vi "Modbus LDO Boolean Decode.vi"(8 "error in":errorcluster, 11 "PLC Data":T1 {"PLC Data - LDO"."Timing"."Absolute Time" format="%<%H:%M:%S%3u>t"; "PLC Data - LDO"."Timing"."Display Time" format="%#.20f"; "PLC Data - LDO"."Timing"."Test Time Ref" format="%#.20f"; "PLC Data - LDO"."Timing"."Precondition Time Ref" format="%#.20f"; "PLC Data - LDO"."Timing"."First Call Time Ref" format="%#.20f"; "PLC Data - FVIR"."Timing"."Absolute Time" format="%<%H:%M:%S%3u>t"; "PLC Data - FVIR"."Timing"."Display Time" format="%#.20f"; "PLC Data - FVIR"."Timing"."Test Time Ref" format="%#.20f"; "PLC Data - FVIR"."Timing"."Precondition Time Ref" format="%#.20f"; "PLC Data - FVIR"."Timing"."First Call Time Ref" format="%#.20f"}) -> (0 "error out":errorcluster, 3 "PLC Data Out":T1 {"PLC Data - LDO"."Timing"."Absolute Time" format="%<%H:%M:%S%3u>t"; "PLC Data - LDO"."Timing"."Display Time" format="%#.20f"; "PLC Data - LDO"."Timing"."Test Time Ref" format="%#.20f"; "PLC Data - LDO"."Timing"."Precondition Time Ref" format="%#.20f"; "PLC Data - LDO"."Timing"."First Call Time Ref" format="%#.20f"; "PLC Data - FVIR"."Timing"."Absolute Time" format="%<%H:%M:%S%3u>t"; "PLC Data - FVIR"."Timing"."Display Time" format="%#.20f"; "PLC Data - FVIR"."Timing"."Test Time Ref" format="%#.20f"; "PLC Data - FVIR"."Timing"."Precondition Time Ref" format="%#.20f"; "PLC Data - FVIR"."Timing"."First Call Time Ref" format="%#.20f"})   [LabVIEW 2023, in "Modbus.lvlib"]
uses:
  Modbus.lvlib
  Modbus PLC Data All.ctl
  Modbus FVIR Control.ctl
  Modbus Timing.ctl
  <vilib>/Utility/miscctls.llb/LVDateTimeRec.ctl
  Modbus LDO Control.ctl
  WritingDataFile/Data to Save.ctl
  support/Terminate Conditions Cluster.ctl
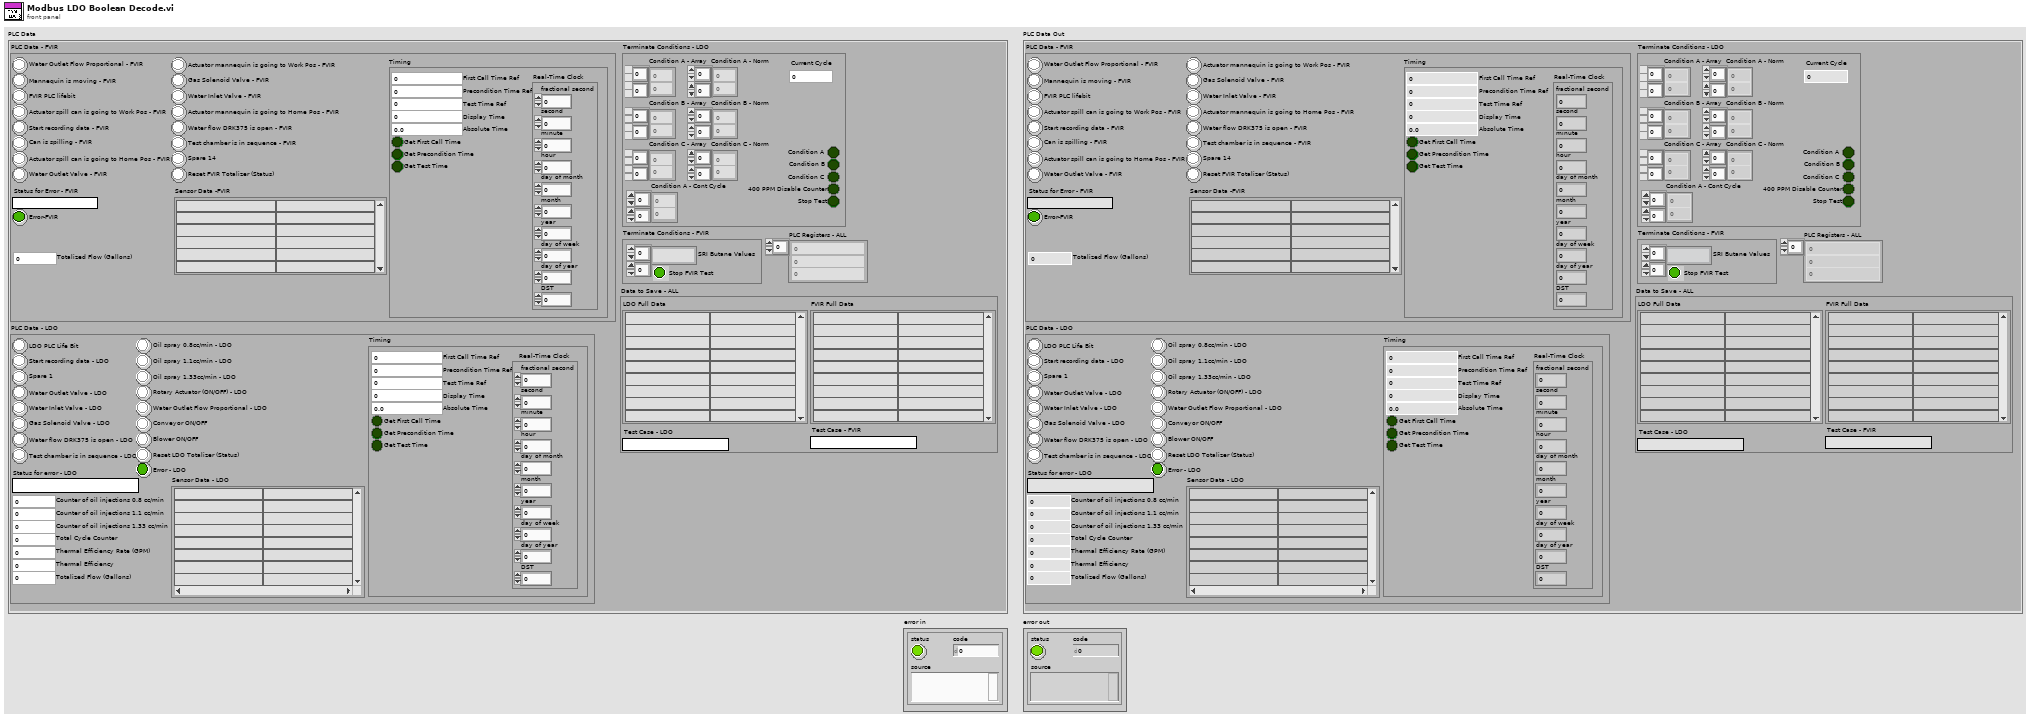
[diagram p1: front panel]
types:
  T1 = typedef "Modbus PLC Data All.ctl" = cluster{"PLC Data - FVIR":T2, "PLC Data - LDO":T5, "PLC Registers - ALL":i16[], "Data to Save - ALL":T6, "Terminate Conditions - LDO":T7, "Terminate Conditions - FVIR":cluster{"SRI Butane Values":string[][], "Stop FVIR Test":bool}}
  T2 = typedef "Modbus FVIR Control.ctl" = cluster{"Reset FVIR Totalizer (Status)":bool, "Spare 14":bool, "Actuator mannequin is going to Work Pos - FVIR":bool, "Actuator mannequin is going to Home Pos - FVIR":bool, "Test chamber is in sequence - FVIR ":bool, "Water flow DRK375 is open - FVIR":bool, "Gas Solenoid Valve - FVIR":bool, "Water Inlet Valve - FVIR":bool, "Water Outlet Flow Proportional - FVIR":bool, "Start recording data - FVIR":bool, "Actuator spill can is going to Work Pos - FVIR":bool, "Actuator spill can is going to Home Pos - FVIR":bool, "Water Outlet Valve - FVIR":bool, "Can is spilling - FVIR":bool, "Mannequin is moving - FVIR":bool, "FVIR PLC lifebit":bool, "Status for Error - FVIR":string, "Error-FVIR":bool, "Sensor Data -FVIR":string[][], "Totalized Flow (Gallons)":dbl, "Timing":T3}
  T3 = typedef "Modbus Timing.ctl" = cluster{"First Call Time Ref":dbl, "Precondition Time Ref":dbl, "Test Time Ref":dbl, "Get First Call Time":bool, "Get Precondition Time":bool, "Get Test Time":bool, "Display Time":dbl, "Real-Time Clock":T4, "Absolute Time":dbl}
  T4 = typedef "LVDateTimeRec.ctl" = cluster{"fractional second":dbl, "second":i32, "minute":i32, "hour":i32, "day of month":i32, "month":i32, "year":i32, "day of week":i32, "day of year":i32, "DST":i32}
  T5 = typedef "Modbus LDO Control.ctl" = cluster{"LDO PLC Life Bit":bool, "Start recording data - LDO":bool, "Spare 1":bool, "Water Outlet Valve - LDO":bool, "Water Inlet Valve - LDO":bool, "Gas Solenoid Valve - LDO":bool, "Water flow DRK375 is open - LDO":bool, "Test chamber is in sequence - LDO":bool, "Oil spray 0.8cc/min - LDO":bool, "Oil spray 1.1cc/min - LDO":bool, "Oil spray 1.33cc/min - LDO":bool, "Rotary Actuator (ON/OFF) - LDO":bool, "Water Outlet Flow Proportional - LDO":bool, "Conveyor ON/OFF":bool, "Blower ON/OFF":bool, "Reset LDO Totalizer (Status)":bool, "Status for error - LDO":string, "Error - LDO":bool, "Sensor Data - LDO":string[][], "Thermal Efficiency Rate (GPM)":dbl, "Thermal Efficiency":dbl, "Totalized Flow (Gallons)":dbl, "Counter of oil injections 1.33 cc/min":u16, "Total Cycle Counter":u16, "Counter of oil injections 1.1 cc/min":u16, "Counter of oil injections 0.8 cc/min":u16, "Timing":T3}
  T6 = typedef "Data to Save.ctl" = cluster{"LDO Full Data":string[][], "FVIR Full Data":string[][], "Test Case - FVIR":string, "Test Case - LDO":string}
  T7 = typedef "Terminate Conditions Cluster.ctl" = cluster{"Condition B - Array":dbl[][], "Current Cycle":u16, "Condition C - Array":dbl[][], "Condition A - Array":dbl[][], "400 PPM Disable Counter":bool, "Condition A - Norm":dbl[][], "Condition B - Norm":dbl[][], "Condition C - Norm":dbl[][], "Condition A":bool, "Condition B":bool, "Condition C":bool, "Condition A - Cont Cycle":dbl[][], "Stop Test":bool}
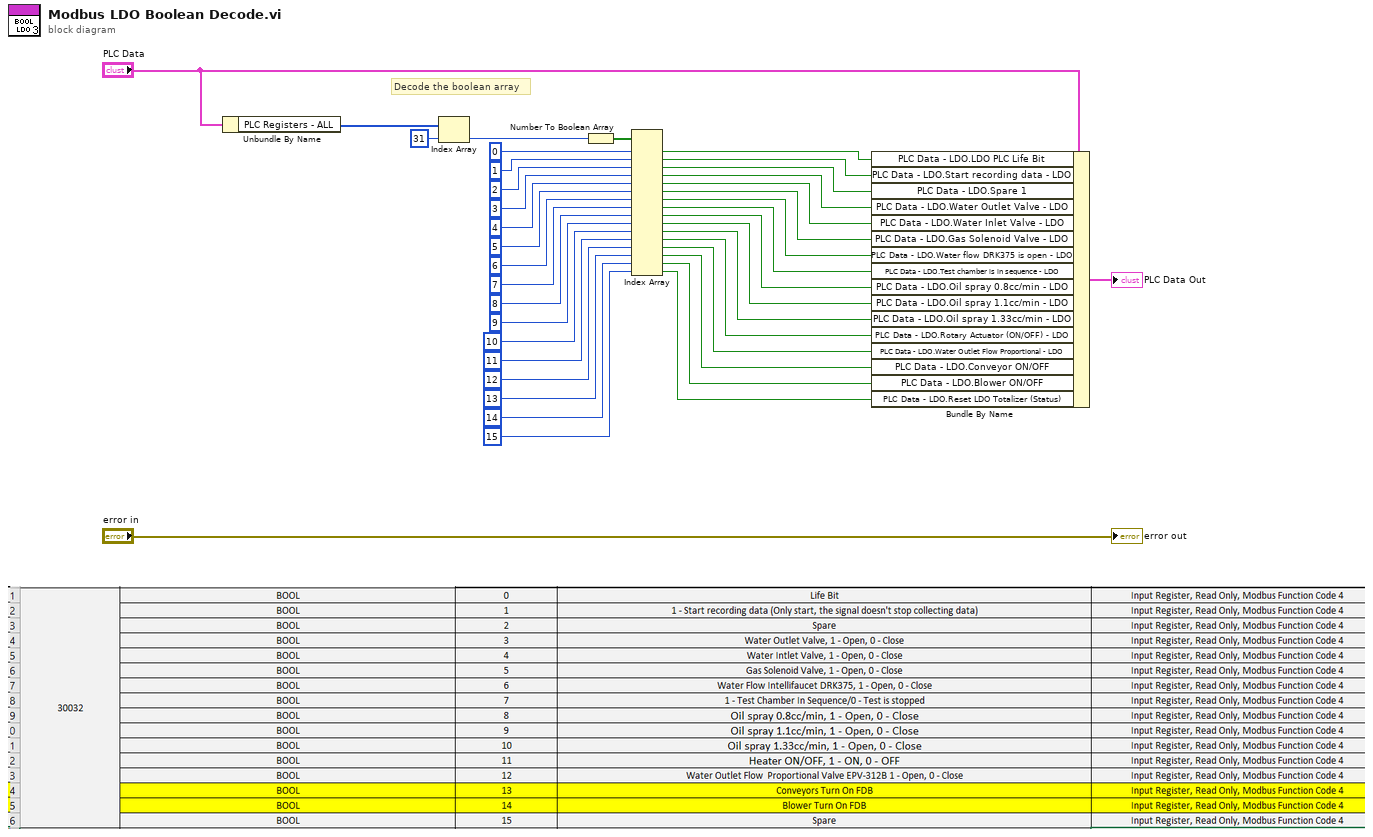
[diagram p0: block diagram]
diagram:
  # "Decode the boolean array"
  n1 = Unbundle By Name("PLC Data") -> ("PLC Registers - ALL"=w2:i16[])
  n2 = Index Array(array=w2, index=31) -> (element=w39:i16)
  n3 = Number To Boolean Array(number=w39) -> (Boolean array=w38:bool[])
  n4 = Index Array(array=w38, index #1=0 ("index"), index #2=1 ("index"), index #3=2 ("index"), index #4=3 ("index"), index #5=4 ("index"), index #6=5 ("index"), index #7=6 ("index"), index #8=7 ("index"), index #9=8 ("index"), index #10=9 ("index"), index #11=10 ("index"), index #12=11 ("index"), index #13=12 ("index"), index #14=13 ("index"), index #15=14 ("index"), index #16=15 ("index")) -> (element #1=w20:bool, element #2=w19:bool, element #3=w18:bool, element #4=w17:bool, element #5=w16:bool, element #6=w15:bool, element #7=w14:bool, element #8=w13:bool, element #9=w12:bool, element #10=w11:bool, element #11=w10:bool, element #12=w9:bool, element #13=w8:bool, element #14=w7:bool, element #15=w6:bool, element #16=w5:bool)
  n5 = Bundle By Name(cluster="PLC Data", "PLC Data - LDO.LDO PLC Life Bit"=w20, "PLC Data - LDO.Start recording data - LDO"=w19, "PLC Data - LDO.Spare 1"=w18, "PLC Data - LDO.Water Outlet Valve - LDO"=w17, "PLC Data - LDO.Water Inlet Valve - LDO"=w16, "PLC Data - LDO.Gas Solenoid Valve - LDO"=w15, "PLC Data - LDO.Water flow DRK375 is open - LDO"=w14, "PLC Data - LDO.Test chamber is in sequence - LDO"=w13, "PLC Data - LDO.Oil spray 0.8cc/min - LDO"=w12, "PLC Data - LDO.Oil spray 1.1cc/min - LDO"=w11, "PLC Data - LDO.Oil spray 1.33cc/min - LDO"=w10, "PLC Data - LDO.Rotary Actuator (ON/OFF) - LDO"=w9, "PLC Data - LDO.Water Outlet Flow Proportional - LDO"=w8, "PLC Data - LDO.Conveyor ON/OFF"=w7, "PLC Data - LDO.Blower ON/OFF"=w6, "PLC Data - LDO.Reset LDO Totalizer (Status)"=w5) -> (→"PLC Data Out":T1)
  "error out" <- "error in"
